vi "Wait Return.vi"(8 "entrée d'erreur (pas d'erreur)":errorcluster, 10 "Property:Data en entrée":string, 11 "Class Instrument (Default) en entrée":refnum<class "Class Instrument (Default).lvclass">) -> (0 "sortie d'erreur":errorcluster, 1 "Return":bool, 2 "Data":string, 3 "Class Instrument (Default) en sortie":refnum<class "Class Instrument (Default).lvclass">, 4 "Status":string)   [LabVIEW 2020, in "Library Test.lvlib" / "P2056_Send_Command_UART.lvclass"]
uses:
  P2056_Send_Command_UART.lvclass
  Instrument/Instrument (Default)/Class Instrument (Default).lvclass
  JSON API/JSON Value/Set from JSON string.vi
  JSON API/JSON Value/JSON Value.lvclass
  P2056_Send_Command_UART.lvclass/P2056_Send_Command_UART.ctl
  JSON API/Variant JSON/Variant JSON.lvlib
  JSON API/Get Polymorphic/JSON GetSet.lvlib
  Commun VI/Library Commun.lvlib
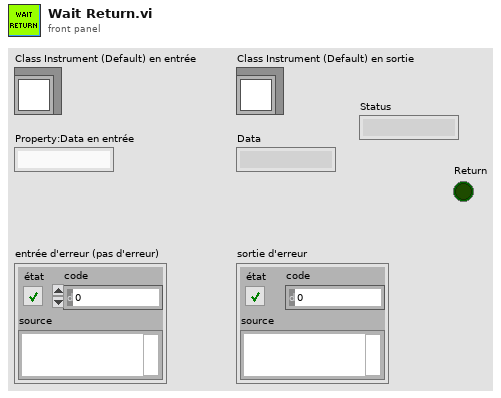
[diagram p1: front panel]
types:
  T1 = cluster{"Frame Read":string, "Frame received":bool, "Frame NOk":bool}
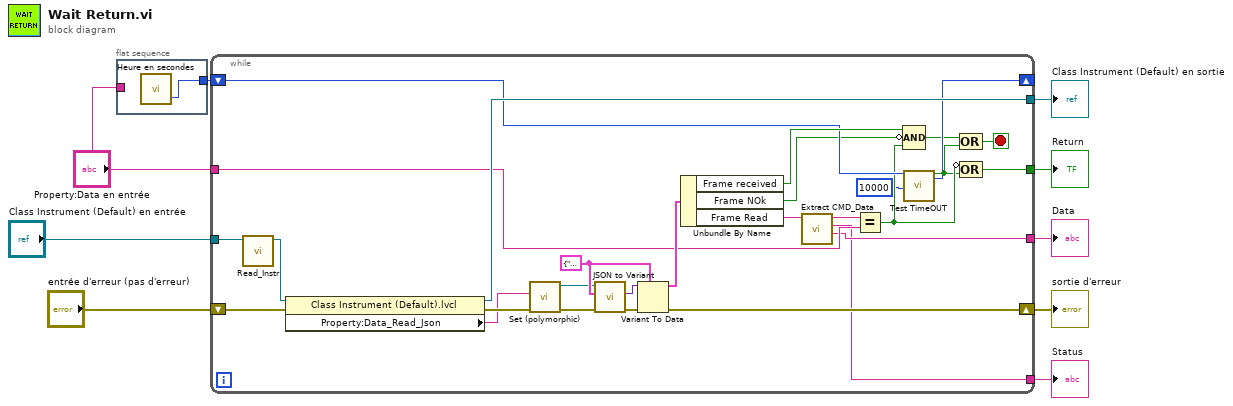
[diagram p0: block diagram]
diagram:
  n1 = flat-sequence {
    tunnel: [w10] -> w8
    tunnel: "Property:Data en entrée" -> [_]
    frame #0 {
      n2 = call "Heure en secondes.vi"() -> ("Heure en milisecondes"=w10:u32)  [unwired: 2 in, 1 out]
    }
  }
  n3 = while {
    tunnel: "Class Instrument (Default) en entrée" -> [w29]
    shift-right: [w16] -> w6
    shift-left: "entrée d'erreur (pas d'erreur)" -> [w14]
    tunnel: [w27] -> w7
    shift-right: [w25] -> _
    shift-left: w8 -> [w26]
    tunnel: [w17] -> w9
    tunnel: "Property:Data en entrée" -> [w23]
    tunnel: [w18] -> w3
    tunnel: [w15] -> w2
    stop <- w12 stop-if-true
    w37 = T1 {"Frame Read"="", "Frame received"=FALSE, "Frame NOk"=FALSE}
    n4 = call-dynamic "Read_Instr.vi"("Class Instrument (Default) en entrée"=w29) -> ("Class Instrument (Default) en sortie"=w30:refnum<class "Class Instrument (Default).lvclass">)  [unwired: 9 in, 1 out]
    n5 = property class="Class Instrument (Default).lvcl"(reference=w30, error in=w14) -> (reference out=w27:refnum<class "Class Instrument (Default).lvclass">, error out=w35:errorcluster, "Property:Data_Read_Json"=w34:string)
    n6 = call-poly "Set (polymorphic).vi"("error in (no error)"=w35, "JSON stream"=w34) -> ("error out"=w31:errorcluster, "JSON Value out"=w33:refnum<class "JSON Value.lvclass">)  [unwired: 7 in, 1 out]
    n7 = call "JSON to Variant.vi"("error in (no error)"=w31, "Variant (Data Type)"=w37, "JSON Value"=w33) -> ("error out"=w32:errorcluster, "Variant out"=w36:variant)  [unwired: 7 in]
    n8 = Variant To Data(error in=w32, type=w37, Variant=w36) -> (data=w38:T1, error out=w16:errorcluster)
    n9 = Unbundle By Name(w38) -> ("Frame received"=w28:bool, "Frame NOk"=w24:bool, "Frame Read"=w21:string)
    n10 = call "Extract CMD_Data.vi"("Frame"=w21) -> ("DATA"=w17:string, "Status"=w15:string, "CMD"=w20:string)  [unwired: 8 in]
    n11 = Equal?(x=w20, y=w23) -> (x = y?=w22:bool)
    n12 = Compound Arithmetic op=AND ("Opérateur arithmétique")(w28, invert w24, w22) -> (w13:bool)
    n13 = call "Test TimeOUT.vi"("OLD Time"=w26, "TimeOut ms"=u32 10000) -> ("Timeout ?"=w11:bool, "NEW Time"=w25:u32)  [unwired: 13 in, 3 out]
    n14 = Compound Arithmetic op=OR ("Opérateur arithmétique")(w13, w11) -> (w12:bool)
    n15 = Compound Arithmetic op=OR ("Opérateur arithmétique")(invert w22, w11) -> (w18:bool)
  }
  "Data" <- w9
  "Class Instrument (Default) en sortie" <- w7
  "sortie d'erreur" <- w6
  "Return" <- w3
  "Status" <- w2
